vi "Driving PID.vi"(8 "Manual Speed":dbl, 9 "Use Distance?":bool, 10 "Setpoint Angle":dbl, 11 "Setpoint Distance":dbl) -> (0 "Encoder Distance":dbl, 1 "Driving Output":dbl(knob) scale=-0.5..0.5, 2 "Turning Output":dbl(knob) scale=-0.5..0.5, 3 "Gyro Angle":dbl(knob) scale=-10.0..10.0, 4 "Boolean Output":bool, 5 "PID Data":T1)   [LabVIEW 2014]
uses:
  <vilib>/addons/control/pid/pid.llb/PID Structure.ctl
  <vilib>/Rock Robotics/WPI/RobotDrive/WPI_RobotDriveGetSetRefNum.vi
  <vilib>/addons/control/pid/pid.llb/PID Control Input Filter (DBL).vi
  <vilib>/addons/control/pid/pid.llb/PID (DBL).vi
  <vilib>/addons/control/pid/pid.llb/PID Structure Conversion (DBL).vi
  <vilib>/addons/control/pid/NI_PID_pid.lvlib
panel:
  out "At Angle":bool
  out "Turning Graph":dbl(graph)
  out "error Graph":dbl(graph)
  out "At Distance":bool
  in  "Driving PID gains":T2={"proportional gain (Kc)"=0.01, "integral time (Ti, min)"=0.0, "derivative time (Td, min)"=0.0}
  in  "Turning PID gains":T2={"proportional gain (Kc)"=0.01, "integral time (Ti, min)"=0.0, "derivative time (Td, min)"=0.0}
  # "3\n.01\n0"
  # ".8\no\n.001"
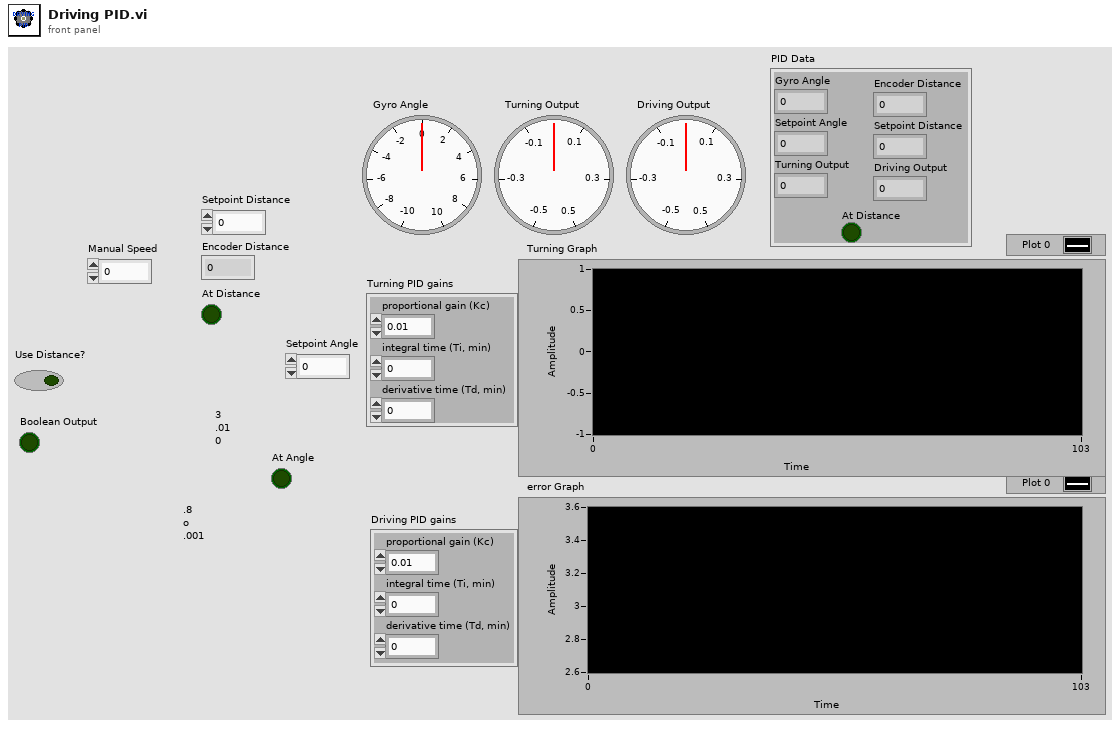
[diagram p1: front panel]
types:
  T1 = cluster{"Gyro Angle":dbl, "Setpoint Angle":dbl, "Turning Output":dbl, dbl, "Setpoint Distance":dbl, "Driving Output":dbl, bool}
  T2 = cluster{"proportional gain (Kc)":dbl, "integral time (Ti, min)":dbl, "derivative time (Td, min)":dbl}
  T3 = typedef "NI_PID_pid.lvlib/PID Structure.ctl" = u16
  T4 = typedef "WPI_EncoderDevRef.ctl" = cluster{"DevStatus":errorcluster, "EncoderIndex":T5, "CounterIndex":T6, "DistancePerCount":dbl, "Decoding Type":T7}
  T5 = typedef "FPGA_EncoderIdx.ctl" = enum8{"Enc 0", "Enc 1", "Enc 2", "Enc 3", "Enc 4", "Enc 5", "Enc 6", "Enc 7", "Invalid"}
  T6 = typedef "FPGA_CounterCtrSystemIndex.ctl" = enum8{"Ctr 0", "Ctr 1", "Ctr 2", "Ctr 3", "Ctr 4", "Ctr 5", "Ctr 6", "Ctr 7", "Invalid"}
  T7 = typedef "WPI_EncoderType.ctl" = enum16{"1x", "2x", "4x"}
  T8 = typedef "WPI_GyroDevRef.ctl" = cluster{"DevStatus":errorcluster, "Analog Module":T9, "Analog Channel":T10, "Offset":dbl, "Gain (VoltsPerDegree/Second)":dbl}
  T9 = typedef "FPGA_TypedefAnalogModule.ctl" = enum16{"Controller 1"}
  T10 = typedef "FPGA_AIChannel.ctl" = enum8{"AI 0", "AI 1", "AI 2", "AI 3", "AI MXP 0", "AI MXP 1", "AI MXP 2", "AI MXP 3", "Invalid"}
  T11 = typedef "WPI_RobotDriveDevRef.ctl" = cluster{"DevStatus":errorcluster, "Motors[]":T12[], "Square Inputs":bool, "Max Output":dbl}
  T12 = typedef "WPI_MotorControlDeviceRef.ctl" = cluster{"DeviceStatus":errorcluster, "Type":T13, "PWM":cluster{"Controller":T14, "PWM Channel":T15, "DeadBand":T16}, "CAN":cluster{"Device Number":u8, "Control Mode":T17, "Semaphore":T18, "Max Vout":dbl, "TalonSRX Control Mode":T19}, "Invert":bool, "TransformRef":T20, "InvTransformRef":T20}
  T13 = typedef "WPI_MotorControlType.ctl" = enum16{"PWM", "CAN", "CANTalonSRX"}
  T14 = typedef "FPGA_TypedefDigitalModule.ctl" = enum16{"Controller 1"}
  T15 = typedef "FPGA_DIOPWMChannel.ctl" = enum8{"PWM 0", "PWM 1", "PWM 2", "PWM 3", "PWM 4", "PWM 5", "PWM 6", "PWM 7", "PWM 8", "PWM 9", "PWM MXP 0", "PWM MXP 1", "PWM MXP 2", "PWM MXP 3", "PWM MXP 4", "PWM MXP 5", "PWM MXP 6", "PWM MXP 7", "PWM MXP 8", "PWM MXP 9", "Invalid"}
  T16 = typedef "WPI_PWMDeadband.ctl" = cluster{"Name":string, "maxPositivePwm":i32, "minPositivePwm":i32, "centerPwm":i32, "maxNegativePwm":i32, "minNegativePwm":i32, "angularRange":u16}
  T17 = typedef "WPI_CANJaguar_ControlMode.ctl" = enum8{"Percent VBus", "Current", "Speed", "Position", "Voltage"}
  T18 = typedef "Semaphore RefNum" = refnum<k1>
  T19 = typedef "WPI_CANTalonSRX_APIControlMode.ctl" = enum8{"Percent VBus", "Speed", "Position", "Slave", "Unchanged / Invalid"}
  T20 = typedef "WPI_PWMTransform_ConPane.ctl" = refnum<vi>
  T21 = cluster{"output":dbl, "Setpoint Angle":dbl, "output":dbl, dbl, "Setpoint Distance":dbl, dbl, bool}
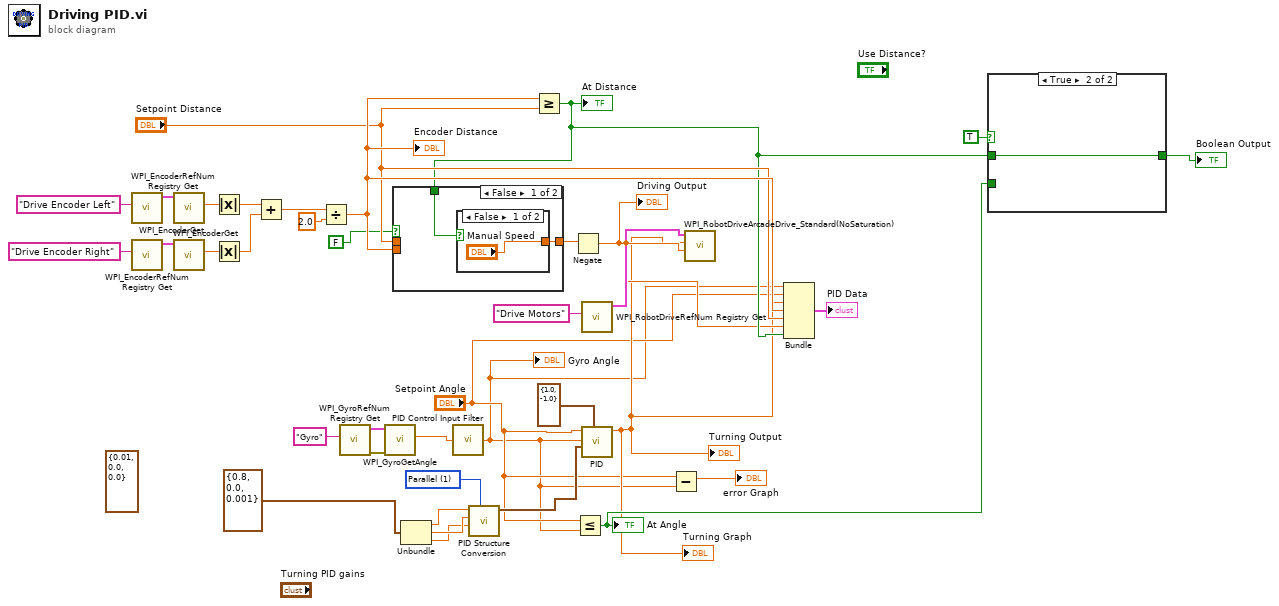
[diagram p0: block diagram]
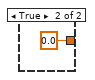
[diagram p3: hidden frame]
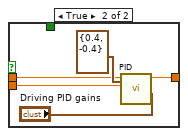
[diagram p4: hidden frame]
diagram:
  w10 = T3 1 items=["Academic (Standard)", "Parallel", "Series"] ("PID structure")
  (unwired) T2 {"proportional gain (Kc)"=0.01, "integral time (Ti, min)"=0.0, "derivative time (Td, min)"=0.0} ("PID gains")
  n1 = call <vilib>:"WPI_EncoderRefNum Registry Get.vi"("refnum name"="Drive Encoder Left") -> ("EncoderDevRef"=w24:T4)  [unwired: 9 in, 1 out]
  n2 = call <vilib>:"WPI_EncoderRefNum Registry Get.vi"("refnum name"="Drive Encoder Right") -> ("EncoderDevRef"=w23:T4)  [unwired: 9 in, 1 out]
  n3 = call <vilib>:"WPI_EncoderGet.vi"("EncoderDevRef"=w24) -> ("Distance"=w30:dbl)  [unwired: 5 in, 5 out]
  n4 = call <vilib>:"WPI_EncoderGet.vi"("EncoderDevRef"=w23) -> ("Distance"=w29:dbl)  [unwired: 5 in, 5 out]
  n5 = Absolute Value(x=w30) -> (abs(x)=w31:dbl)
  n6 = Absolute Value(x=w29) -> (abs(x)=w32:dbl)
  n7 = Add(x=w31, y=w32) -> (x+y=w27:dbl)
  n8 = Divide(x=w27, y=2.0) -> (x/y=w22:dbl)
  "Encoder Distance" <- w22
  n9 = call <vilib>:"WPI_GyroRefNum Registry Get.vi"("refnum name"="Gyro") -> ("error out"=w35:errorcluster, "GyroDevRef"=w36:T8)  [unwired: 9 in]
  n10 = call <vilib>:"WPI_GyroGetAngle.vi"("error in (no error)"=w35, "GyroDevRef"=w36) -> ("Angle"=w5:dbl)  [unwired: 6 in, 3 out]
  n11 = Unbundle(T2 {"proportional gain (Kc)"=0.8, "integral time (Ti, min)"=0.0, "derivative time (Td, min)"=0.001} ("PID gains")) -> ("proportional gain (Kc)"=w8:dbl, "integral time (Ti, min)"=w7:dbl, "derivative time (Td, min)"=w6:dbl)
  n12 = call-poly <vilib>:"PID Control Input Filter.vi"("input"=w5) -> ("output"=w3:dbl)  [unwired: 4 in]
  "Gyro Angle" <- w3
  n13 = call-poly <vilib>:"PID Structure Conversion.vi"("PID structure"=w10, "derivative"=w6, "integral"=w7, "proportional"=w8) -> ("PID gains"=w9:T2)  [unwired: 7 in]
  n14 = Greater Or Equal?(x=w22, y="Setpoint Distance") -> (x >= y?=w17:bool)
  "At Distance" <- w17
  n15 = case shown="False" FALSE {
    tunnel: w22 -> [_ w44]
    tunnel: "Setpoint Distance" -> [_ w43]
    tunnel: [w38 w42] -> w18
    tunnel: w17 -> [w39 _]
    frame False {
      n16 = case shown="False" w39 {
        tunnel: ["Manual Speed" 0.0 ("Manual Speed")] -> w38
        frame False {
        }
        frame True {
        }
      }
    }
    frame True {
      n17 = call-poly <vilib>:"PID.vi"("output range"=cluster{"output high":dbl, "output low":dbl} {"output high"=0.4, "output low"=-0.4}, "PID gains"="Driving PID gains", "process variable"=w44, "setpoint"=w43) -> ("output"=w42:dbl)  [unwired: 6 in, 1 out]
    }
  }
  n18 = Negate(x=w18) -> (-x=w13:dbl)
  "Driving Output" <- w13
  n19 = Less Or Equal?(x="Setpoint Angle", y=w3) -> (x <= y?=w15:bool)
  "At Angle" <- w15
  n20 = call <vilib>:"WPI_RobotDriveRefNum Registry Get.vi"("refnum name"="Drive Motors") -> ("RobotDriveDevRef"=w14:T11)  [unwired: 1 in, 9 out]
  n21 = call-poly <vilib>:"PID.vi"("output range"=cluster{"output high":dbl, "output low":dbl} {"output high"=1.0, "output low"=-1.0}, "PID gains"=w9, "process variable"=w3, "setpoint"="Setpoint Angle") -> ("output"=w12:dbl)  [unwired: 6 in, 1 out]
  "Turning Output" <- w12
  "Turning Graph" <- w12
  n22 = Subtract(x="Setpoint Angle", y=w3) -> (x-y=→"error Graph":dbl)
  n23 = call <vilib>:"WPI_RobotDriveArcadeDrive_Standard(NoSaturation).vi"("Y axis value"=w13, "X axis value"=w12, "RobotDriveDevRef"=w14) -> ()  [unwired: 1 in, 8 out]
  n24 = Bundle("output"=w3, "Setpoint Angle"="Setpoint Angle", "output"=w12, w22, "Setpoint Distance"="Setpoint Distance", w13, w17) -> (→"PID Data":T21)  [unwired: 1 in]
  n25 = case shown="True" TRUE {
    tunnel: w17 -> [_ w48]
    tunnel: [w47 w48] -> w16
    tunnel: w15 -> [w47 _]
    frame False {
    }
    frame True {
    }
  }
  "Boolean Output" <- w16
